vi "DriveCommandToMotorPower.vi"(8 "Drive Command Override":bool, 9 "Drive Command Override (ul) [-1,1]":dbl, 10 "Drive Command (ul) [-1,1]":dbl, 11 "Actual Shifter State":T1(ring)) -> (2 "Motor Power (ul) [-1,1]":dbl)   [LabVIEW 2020]
doc: "This VI linearizes the the drive motor behavior by converting the linear, unitless drive command to the appropriate drive motor power. Handles low and high gear shifter states. The motors shoulds be calibrated with voltage compensation switched ON."
uses:
  GlobalDrivebase.vi
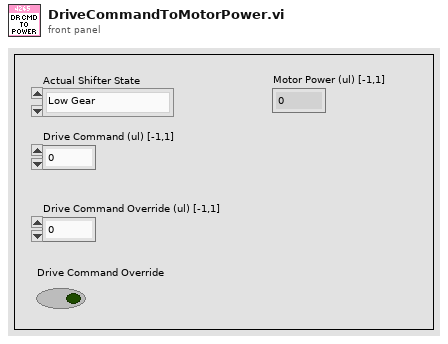
[diagram p1: front panel]
types:
  T1 = enum16{"Low Gear", "High Gear", "Transiting", "Unknown", "Force Low Gear"}
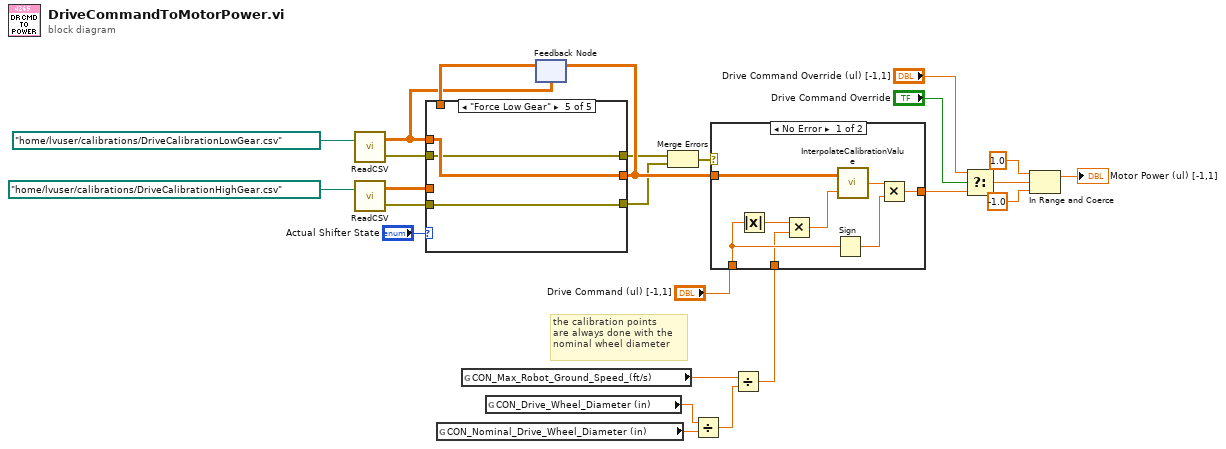
[diagram p0: block diagram]
diagram:
  # "the calibration points\nare always done with the \nnominal wheel diameter"
  n1 = call "ReadCSV.vi"("File Path (.csv)"=path "/home/lvuser/calibrations/DriveCalibrationLowGear.csv" ("path")) -> ("File Open Eror"=w18:errorcluster, "Data (index by row)"=w19:dbl[][])  [unwired: 1 in]
  n2 = call "ReadCSV.vi"("File Path (.csv)"=path "/home/lvuser/calibrations/DriveCalibrationHighGear.csv" ("path")) -> ("File Open Eror"=w16:errorcluster, "Data (index by row)"=w20:dbl[][])  [unwired: 1 in]
  n3 = global read "GlobalDrivebase.vi" "CON_Nominal_Drive_Wheel_Diameter (in)"() -> (w5:dbl)
  n4 = global read "GlobalDrivebase.vi" "CON_Max_Robot_Ground_Speed_(ft/s)"() -> (w3:dbl)
  n5 = global read "GlobalDrivebase.vi" "CON_Drive_Wheel_Diameter (in)"() -> (w4:dbl)
  n6 = feedback #1(w19) -> (w21:dbl[][])
  n7 = case shown="\"Force Low Gear\"" "Actual Shifter State" {
    tunnel: w20 -> [_ w31 _ _ _]
    tunnel: w19 -> [w28 _ _ _ w40]
    tunnel: [w28 w31 w34 w37 w40] -> w22
    tunnel: w21 -> [_ _ w34 w37 _]
    tunnel: [w27 w30 w33 w36 w39] -> w17
    tunnel: w18 -> [w27 w30 w33 w36 w39]
    tunnel: [w26 w29 w32 w35 w38] -> w15
    tunnel: w16 -> [w26 w29 w32 w35 w38]
    frame "Low Gear", Default {
    }
    frame "High Gear" {
    }
    frame "Transiting" {
    }
    frame "Unknown" {
    }
    frame "Force Low Gear" {
    }
  }
  n8 = feedback-in #1(w22) -> ()
  n9 = Merge Errors(w17, w15) -> (w14:errorcluster)
  n10 = Divide(x=w4, y=w5) -> (x/y=w2:dbl)
  n11 = Divide(x=w3, y=w2) -> (x/y=w1:dbl)
  n12 = case shown="No Error" w14 {
    tunnel: "Drive Command (ul) [-1,1]" -> [w46 w49]
    tunnel: [w43 w49] -> w12
    tunnel: w22 -> [w42 _]
    tunnel: w1 -> [w41 _]
    frame No Error {
      n13 = Absolute Value(x=w46) -> (abs(x)=w47:dbl)
      n14 = Multiply(x=w47, y=w41) -> (x*y=w48:dbl)
      n15 = Sign(1:w46) -> (0:w44:dbl)
      n16 = call "InterpolateCalibrationValue.vi"("Input"=w48, "Calibration Data"=w42) -> ("Interpolated Output"=w45:dbl)
      n17 = Multiply(x=w45, y=w44) -> (x*y=w43:dbl)
    }
    frame Error {
    }
  }
  n18 = Select(t="Drive Command Override (ul) [-1,1]", s="Drive Command Override", f=w12) -> (s? t:f=w9:dbl)
  n19 = In Range and Coerce(upper limit=1.0, x=w9, lower limit=-1.0) -> (coerced(x)=→"Motor Power (ul) [-1,1]":dbl)  [unwired: 1 out]
